vi "Choreo_TrajectorySwerve_GetTotalTime.vi"(11 "ChoreoTrajectorySwerve":T1) -> (3 "TotalTime":dbl)   [LabVIEW 2019, in "ChoreoLib.lvlib"]
doc: "Return total time duration of this trajectory\n\nInputs: \n - ChoreoTrajectory - cluster - Input trajectory\n\nOutputs:\n - TotalTime - double - The total time duration of this trajectory.\n."
uses:
  ChoreoLib.lvlib
  TypeDef/ChoreoTrajectorySwerve.ctl
  TypeDef/ChoreoSwerveSample.ctl
  TypeDef/ChoreoEventMarker.ctl
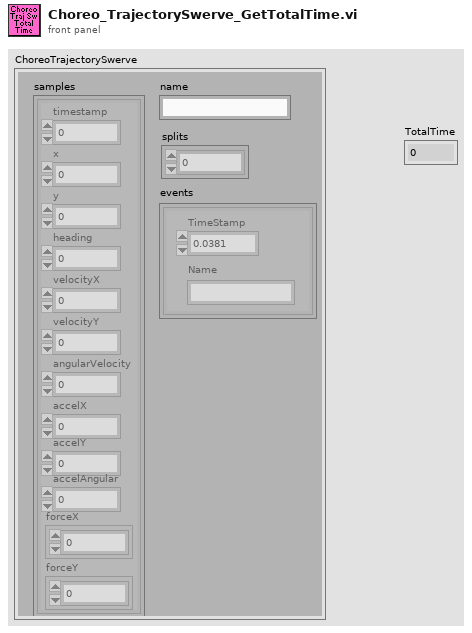
[diagram p1: front panel]
types:
  T1 = typedef "ChoreoLib.lvlib/ChoreoTrajectorySwerve.ctl" = cluster{"name":string, "samples":T2[], "splits":i32[], "events":T3[]}
  T2 = typedef "ChoreoLib.lvlib/ChoreoSwerveSample.ctl" = cluster{"timestamp":dbl, "x":dbl, "y":dbl, "heading":dbl, "velocityX":dbl, "velocityY":dbl, "angularVelocity":dbl, "accelX":dbl, "accelY":dbl, "accelAngular":dbl, "forceX":dbl[], "forceY":dbl[]}
  T3 = typedef "ChoreoLib.lvlib/ChoreoEventMarker.ctl" = cluster{"TimeStamp":dbl, "Name":string}
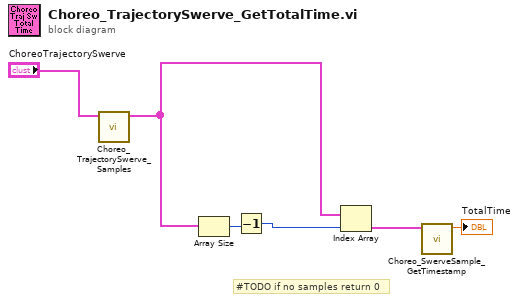
[diagram p0: block diagram]
diagram:
  # "#TODO if no samples return 0"
  n1 = call "Choreo_TrajectorySwerve_Samples.vi"("ChoreoTrajectorySwerve"="ChoreoTrajectorySwerve") -> ("samples"=w1:T2[])  [unwired: 10 in]
  n2 = Array Size(array=w1) -> (size(s)=w6:i32)
  n3 = Decrement(x=w6) -> (x-1=w5:i32)
  n4 = Index Array(array=w1, index=w5) -> (element=w4:T2)
  n5 = call "Choreo_SwerveSample_GetTimestamp.vi"("ChoreoSwerveSample"=w4) -> ("Timestamp"=→"TotalTime":dbl)  [unwired: 10 in]
